vi "Memory.Pointer.Read.Safe.1D.I64.vi"(8 "error in (no error)":errorcluster, 9 "count":u64 format="%d elements", 10 "buffer in":i64[](array[numeric]), 11 "pointer in":refnum<class "Memory.Pointer.lvclass">) -> (0 "error out":errorcluster, 1 "count out":u64 format="%d elements", 2 "buffer out":i64[](array[numeric]), 3 "pointer out":refnum<class "Memory.Pointer.lvclass">)   [LabVIEW 2016, in "Memory Manager.lvlib" / "Memory.Pointer.lvclass"]
doc: "Reads from the address specified by <b>pointer</b> into <b>value</b>.\n\n<b>Note:</b> This VI is <b>safe</b>.\n\nSafe means that this function evaluates the size parameter of <b>pointer</b> to ensure that is inbounds of allocated memory before peforming a memory read/write. Reading/writing more data to a pointer than it has allocated can corrupt or crash LabVIEW."
uses:
  Memory.Pointer.lvclass
  Memory.Pointer.lvclass/Memory.Pointer.ctl
  Accessors/Get Address.vi
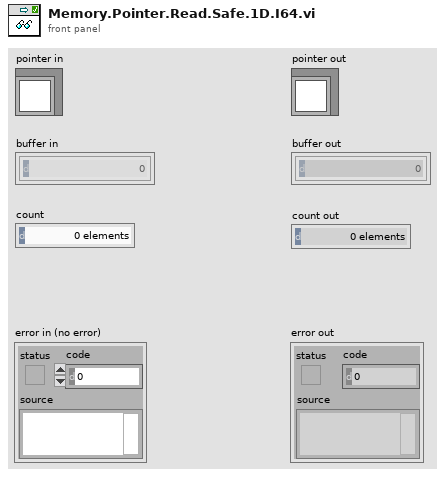
[diagram p1: front panel]
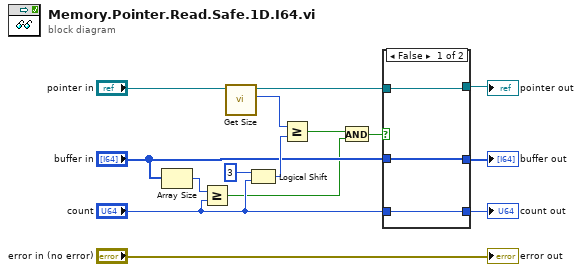
[diagram p0: block diagram]
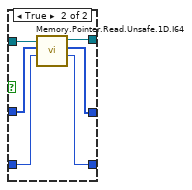
[diagram p2: hidden frame]
diagram:
  n1 = Array Size(array="buffer in") -> (size(s)=w3:i32)
  n2 = Greater Or Equal?(x=w3, y="count") -> (x >= y?=w1:bool)
  n3 = call "Get Size.vi"("Pointer in"="pointer in") -> ("size"=w12:u64, "Pointer out"=w11:refnum<class "Memory.Pointer.lvclass">)  [unwired: 8 in, 1 out]
  n4 = Logical Shift(y=i16 3, x="count") -> (x << y=w13:u64)
  n5 = Greater Or Equal?(x=w12, y=w13) -> (x >= y?=w5:bool)
  n6 = And(x=w5, y=w1) -> (x .and. y?=w6:bool)
  n7 = case shown="False" w6 {
    tunnel: w11 -> [w18 w24]
    tunnel: [w18 w23] -> w10
    tunnel: "buffer in" -> [w17 w22]
    tunnel: "count" -> [w16 w21]
    tunnel: [w16 w20] -> w9
    tunnel: [w17 w19] -> w8
    frame False {
    }
    frame True {
      n8 = call "Memory.Pointer.Read.Unsafe.1D.I64.vi"("count"=w21, "buffer in"=w22, "pointer in"=w24) -> ("count out"=w20:u64, "buffer out"=w19:i64[], "pointer out"=w23:refnum<class "Memory.Pointer.lvclass">)  [unwired: 5 in, 1 out]
    }
  }
  "pointer out" <- w10
  "buffer out" <- w8
  "count out" <- w9
  "error out" <- "error in (no error)"
